vi "Ke2000 Set Current Range.vi"(8 "error in (no error)":errorcluster, 9 "Set CURR Range?":u16(ring) items=["10mA", "100mA", "3A"], 11 "VISA resource name":refnum<visa-resource-name>) -> (0 "error out":errorcluster, 3 "VISA resource name out":refnum<visa-resource-name>)   [LabVIEW 2012]
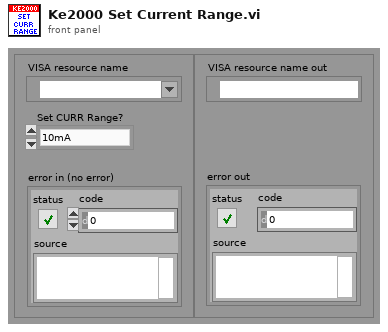
[diagram p1: front panel]
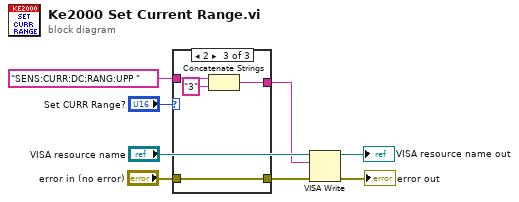
[diagram p0: block diagram]
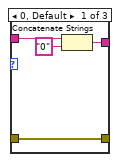
[diagram p2: hidden frame]
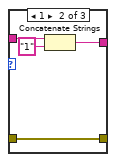
[diagram p3: hidden frame]
diagram:
  n1 = case shown="2" "Set CURR Range?" {
    tunnel: "SENS:CURR:DC:RANG:UPP " ("write buffer") -> [w11 w16 w20]
    tunnel: [w12 w14 w18] -> w4
    tunnel: "error in (no error)" -> [w9 w13 w17]
    tunnel: [w9 w13 w17] -> w2
    frame 0, Default {
      n2 = Concatenate Strings(w11, "0" ("string")) -> (w12:string)
    }
    frame 1 {
      n3 = Concatenate Strings(w16, "1" ("string")) -> (w14:string)
    }
    frame 2 {
      n4 = Concatenate Strings(w20, "3" ("string")) -> (w18:string)
    }
  }
  n5 = VISA Write(VISA resource name="VISA resource name", write buffer=w4, error in (no error)=w2) -> (VISA resource name out=→"VISA resource name out":refnum<visa-resource-name>, error out=→"error out":errorcluster)  [unwired: 1 out]
